vi "FRC Line Tracking.vi"() -> ()   [LabVIEW 2018]
uses:
  source/library/Types/Intersection.ctl
  source/library/Types/Vector.ctl
  <vilib>/Rock Robotics/SystemInterfaces/spilib/spi_bus.ctl
  source/library/Interface/Pixy Com.lvclass
  source/library/Pixy2.lvlib
  source/deviceSupport/FRC/SPI/RoboRIO SPI.lvclass
panel:
  in  "Stop Button":bool
  out "error out":errorcluster
  out "vectors":T1[](array[typedef])
  out "intersections":T2[](array[typedef])
  in  "feature map":u8=7 format="%.0x"
  in  "features":enum16{"Main Features", "All Features"}(ring)
  out "view":picture
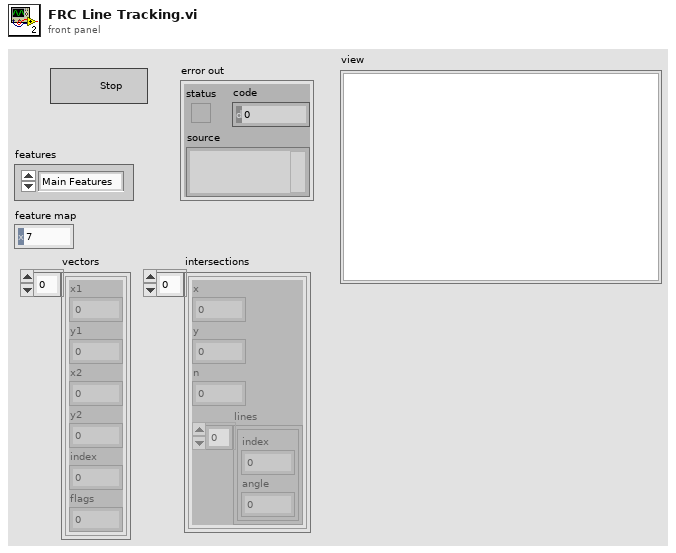
[diagram p1: front panel]
types:
  T1 = typedef "Pixy2.lvlib/Vector.ctl" = cluster{"x1":u8, "y1":u8, "x2":u8, "y2":u8, "index":u8, "flags":u8}
  T2 = typedef "Pixy2.lvlib/Intersection.ctl" = cluster{"x":u8, "y":u8, "n":u8, "lines":cluster{"index":u8, "angle":i16}[]}
  T3 = typedef "spi_bus.ctl" = enum16{"SPI On-Board, CS0", "SPI On-Board, CS1", "SPI On-Board, CS2", "SPI On-Board, CS3", "SPI MXP", "Invalid"}
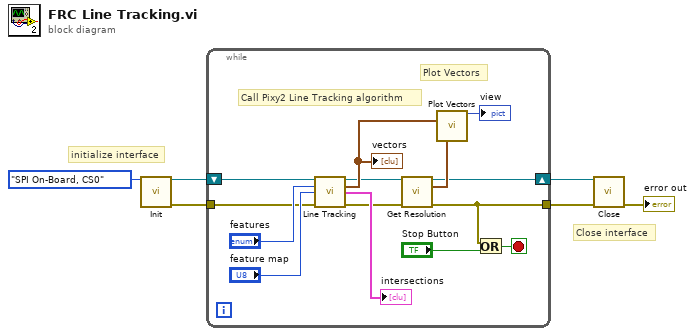
[diagram p0: block diagram]
diagram:
  # "initialize interface"
  # "Close interface"
  n1 = call "Init.vi"("SPI Bus"=spi_bus."SPI On-Board, CS0") -> ("comm interface out"=w2:refnum<class "Pixy Com.lvclass">, "error out"=w1:errorcluster)  [unwired: 13 in]
  n2 = while {
    shift-right: [w12] -> w5
    shift-left: w2 -> [w11]
    tunnel: w1 -> [w10]
    tunnel: [w8] -> w4
    stop <- w7 stop-if-true
    # "Call Pixy2 Line Tracking algorithm"
    # "Plot Vectors"
    n3 = call "Line Tracking.vi"("comm interface in"=w11, "features"="features", "feature map"="feature map", "error in"=w10) -> ("comm interface out"=w16:refnum<class "Pixy Com.lvclass">, "vectors"=w18:T1[], "intersections"=→"intersections":T2[], "error out"=w15:errorcluster)  [unwired: 7 in, 1 out]
    "vectors" <- w18
    n4 = call "Get Resolution.vi"("comm interface in"=w16, "error in"=w15) -> ("comm interface out"=w12:refnum<class "Pixy Com.lvclass">, "resolution"=w14:cluster{"width":u16, "height":u16}, "error out"=w8:errorcluster)  [unwired: 11 in]
    n5 = call "Plot Vectors.vi"("vectors"=w18, "pixy resolution"=w14) -> ("picture out"=→"view":picture)  [unwired: 13 in]
    n6 = Or(x=w8, y="Stop Button") -> (x .or. y?=w7:bool)
  }
  n7 = call-dynamic "Close.vi"("comm interface in"=w5, "error in"=w4) -> ("error out"=→"error out":errorcluster)  [unwired: 13 in]
